vi "Get Channel Group Decimation.vi"(8 "error in":errorcluster, 11 "channel group in":T1 format="%.0x") -> (0 "error out":errorcluster, 2 "decimation":i32=1 min=1, 3 "channel group out":T1 format="%.0x")   [LabVIEW 2027, in "Embedded Data Logger Scripting.lvlib"]
uses:
  Embedded Data Logger Scripting.lvlib
  <vilib>/NI VeriStand/Custom Device API/Custom Device Item Ref.ctl
  Shared/Constants.vi
  <vilib>/NI VeriStand/Custom Device Tools/Custom Device Utility Library/NI VeriStand - Search for Item by GUID.vi
  <vilib>/NI VeriStand/Custom Device Tools/Custom Device Utility Library/Custom Device Utility Library.lvlib
  Shared/Embedded Data Logger Shared.lvlib
  <vilib>/NI VeriStand/Custom Device API/Custom Device API.lvlib
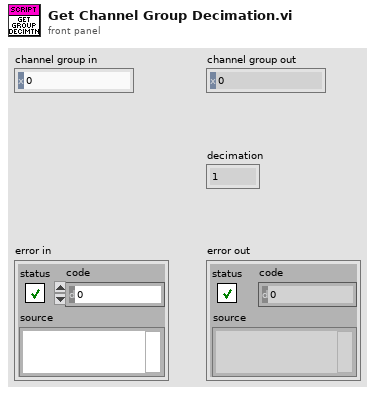
[diagram p1: front panel]
types:
  T1 = typedef "Custom Device API.lvlib/Custom Device Item Ref.ctl" = u64
  T2 = typedef "Custom Device API.lvlib/Custom Device Channel.ctl" = cluster{"Type":T3, "Units":string, "Default Value":dbl, "Faultable":bool, "Scalable":bool}
  T3 = typedef "Custom Device API.lvlib/Custom Device Channel Type.ctl" = enum16{"Input", "Output"}
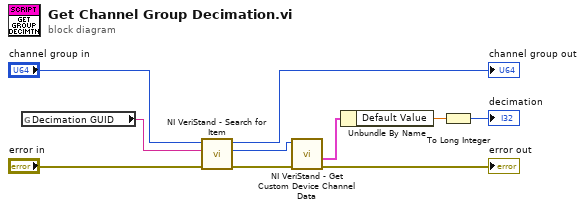
[diagram p0: block diagram]
diagram:
  n1 = global read "Constants.vi" "Decimation GUID"() -> (w10:string)
  n2 = call-poly <vilib>:"NI VeriStand - Search for Item.vi"("error in"="error in", "Item GUID"=w10, "Section Ref in"="channel group in") -> ("error out"=w6:errorcluster, "Item Ref"=w5:T1, "Section Ref out"=→"channel group out":T1)  [unwired: 6 out]
  n3 = call <vilib>:"NI VeriStand - Get Custom Device Channel Data.vi"("error in (no error)"=w6, "Channel Ref in"=w5) -> ("error out"=→"error out":errorcluster, "Channel"=w8:T2)  [unwired: 8 out]
  n4 = Unbundle By Name(w8) -> ("Default Value"=w7:dbl)
  n5 = To Long Integer(number=w7) -> (32bit integer=→"decimation":i32)
